vi "Periodsk utvidelse.vi"(8 "error in (no error)":errorcluster, 9 "Waveform in":waveform(dbl)) -> (0 "error out":errorcluster, 1 "Waveform out":waveform(dbl))   [LabVIEW 2016]
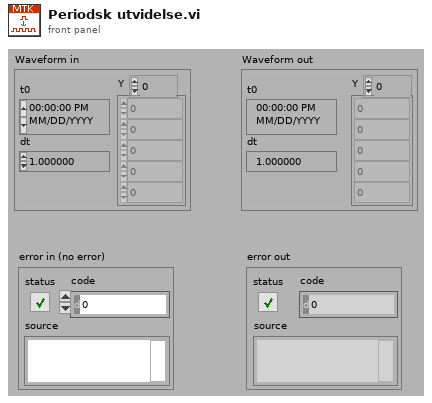
[diagram p1: front panel]
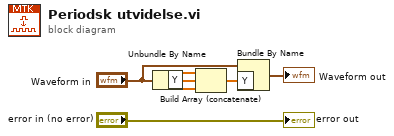
[diagram p0: block diagram]
diagram:
  n1 = Unbundle By Name("Waveform in") -> ("Y"=w2:dbl[])
  n2 = Build Array (concatenate)(w2, w2, w2) -> (w3:dbl[])
  n3 = Bundle By Name(cluster="Waveform in", "Y"=w3) -> (→"Waveform out":waveform(dbl))
  "error out" <- "error in (no error)"
